vi "Truncate I32 to I 16.vi"(11 "Data":i32[](array[numeric]) format="%.0f (%b)") -> (1 "Bits":i32, 2 "divider":i32, 3 "Data out":i16[](array[numeric]) format="%.0f (%b)")   [LabVIEW 2016]
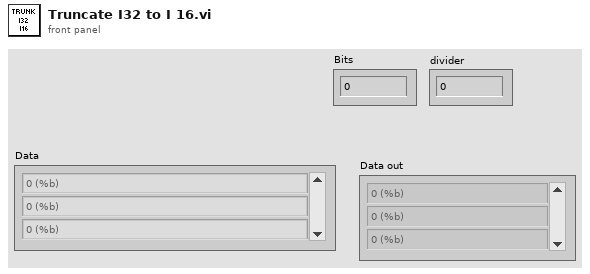
[diagram p1: front panel]
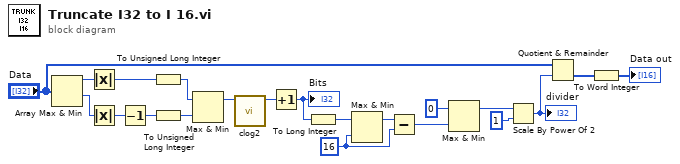
[diagram p0: block diagram]
diagram:
  w12 = 16 ("y")
  n1 = Array Max & Min(array="Data") -> (max value=w20:i32, min value=w21:i32)  [unwired: 2 out]
  n2 = Absolute Value(x=w20) -> (abs(x)=w19:i32)
  n3 = Absolute Value(x=w21) -> (abs(x)=w18:i32)
  n4 = Decrement(x=w18) -> (x-1=w2:i32)
  n5 = To Unsigned Long Integer(number=w19) -> (unsigned 32bit integer=w16:u32)
  n6 = To Unsigned Long Integer(number=w2) -> (unsigned 32bit integer=w15:u32)
  n7 = Max & Min(x=w16, y=w15) -> (max(x,y)=w17:u32)  [unwired: 1 out]
  n8 = call "clog2.vi"("Number"=w17) -> ("clog2"=w10:i32)  [unwired: 10 in]
  n9 = Increment(x=w10) -> (x+1=w3:i32)
  "Bits" <- w3
  n10 = To Long Integer(number=w3) -> (32bit integer=w5:i32)
  n11 = Max & Min(x=w5, y=w12) -> (max(x,y)=w11:i32)  [unwired: 1 out]
  n12 = Subtract(x=w11, y=w12) -> (x-y=w9:i32)
  n13 = Max & Min(x=0, y=w9) -> (max(x,y)=w7:i32)  [unwired: 1 out]
  n14 = Scale By Power Of 2(n=w7, x=1) -> (x*2^n=w6:i32)
  "divider" <- w6
  n15 = Quotient & Remainder(x="Data", y=w6) -> (floor(x/y)=w4:i32[])  [unwired: 1 out]
  n16 = To Word Integer(number=w4) -> (16bit integer=→"Data out":i16[])
